vi "SP Calculate TYY.vi"(10 "SP Array (SXX, SXY, SYX, SYY)":cdb[](array[numeric])) -> (2 "TYY":cdb)   [LabVIEW 2011]
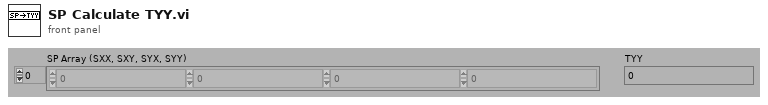
[diagram p1: front panel]
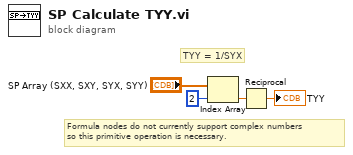
[diagram p0: block diagram]
diagram:
  # "TYY = 1/SYX"
  # "Formula nodes do not currently support complex numbers\nso this primitive operation is necessary."
  n1 = Index Array(array="SP Array (SXX, SXY, SYX, SYY)", index=2) -> (element=w2:cdb)
  n2 = Reciprocal(x=w2) -> (1/x=→"TYY":cdb)
